vi "Save.vi"(8 "error in (no error)":errorcluster, 11 "Test Configs In":T1) -> (0 "error out":errorcluster, 3 "Test Configs Out":T1)   [LabVIEW 2015]
doc: "Save a test configuration XML file to the path chosen."
uses:
  Type Defs/Sequence Parameters Ref.ctl
  <vilib>/Utility/xml.llb/Write to XML File(string).vi
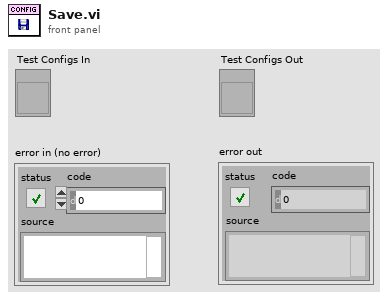
[diagram p1: front panel]
types:
  T1 = typedef "Sequence Parameters Ref.ctl" = refnum<vi>
  T2 = enum16{"open", "replace", "create", "open or create", "replace or create", "replace or create with confirmation"}
  T3 = typedef "Sequence Parameters.ctl" = cluster{"Test Name":string, "Target":T4, "Host IP Address":string, "Target IP Address":string, "Shared Variable Host":enum16{"Target", "Host"}, "Shared Variable Writer":enum16{"Target", "Host"}, "Variable Data Type":T5, "# of Variables per Library":u16, "Update Rate (Hz)":dbl, "Read Rate (Hz)":dbl, "Floor":u32, "Ceiling":u32, "Delta":u32}
  T4 = typedef "Target Type.ctl" = enum16{"cRIO-9012", "cRIO-9014", "cRIO-9022", "cRIO-9023", "cRIO-9024", "cRIO-9025", "cRIO-9068", "cRIO-9073", "cRIO-9074", "cRIO-9075", "cRIO-9076", "cRIO-9081", "cRIO-9082", "myRIO-1900", "myRIO-1950", "PXI-8101", "PXI-8115", "PXI-8119", "PXI-8820", "PXIe-8100", "PXIe-8101", "PXIe-8133", "PXIe-8135", "PXIe-8820", "sbRIO-9605", "sbRIO-9606", "sbRIO-9623", "sbRIO-9626", "sbRIO-9633", "sbRIO-9636", "Unlisted (Linux-RT)", "Unlisted (PharLap)", "Unlisted (VxWorks)", "Windows Target"}
  T5 = typedef "Variable Data Type.ctl" = enum16{"U8", "U16", "U32", "U64", "I8", "I16", "I32", "I64", "Single", "Double", "Boolean", "String"}
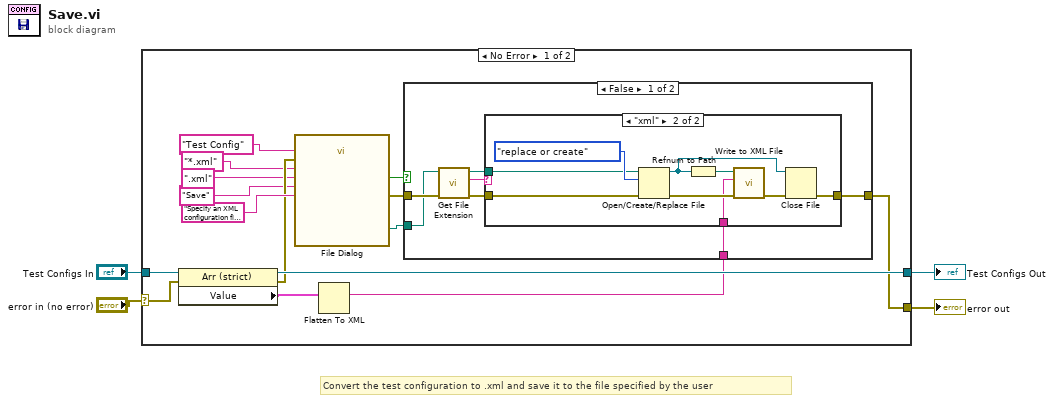
[diagram p0: block diagram]
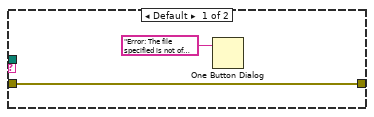
[diagram p2: hidden frame]
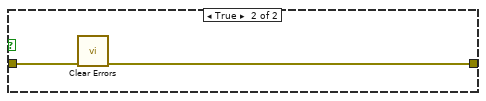
[diagram p3: hidden frame]
diagram:
  # "Convert the test configuration to .xml and save it to the file specified by the user"
  n1 = case shown="No Error" "error in (no error)" {
    selector: "error in (no error)" -> [w18 w40]
    tunnel: "Test Configs In" -> [w19 w41]
    tunnel: [w16 w41] -> w1
    tunnel: [w6 w40] -> w3
    frame No Error {
      n2 = property class="Arr (strict)"(reference=w19, error in=w18) -> (reference out=w16:T1, error out=w13:errorcluster, "Value"=w17:T3[])
      n3 = call "File Dialog"("prompt"="Specify an XML configuration file to create or replace", "button label"="Save", "default name"="Test Config", "error in"=w13, "pattern (all files)"="*.xml", "pattern label"=".xml" ("pattern (all files)")) -> ("selected path"=w10:path, "cancelled"=w12:bool, "error out"=w11:errorcluster)  [unwired: 6 in, 1 out]
      n4 = Flatten To XML(anything=w17) -> (xml string=w5:string)
      n5 = case shown="False" w12 {
        tunnel: w11 -> [w26 w39]
        tunnel: w10 -> [w25 _]
        tunnel: [w21 w38] -> w6
        tunnel: w5 -> [w20 _]
        frame False {
          n6 = call <vilib>:"Get File Extension.vi"("error in (no error)"=w26, "file"=w25) -> ("error out"=w23:errorcluster, "lowercase file extension"=w24:string, "dup file"=w22:path)  [unwired: 5 in, 2 out]
          n7 = case shown="\"xml\"" w24 {
            tunnel: w23 -> [w27 w33]
            tunnel: w22 -> [_ w32]
            tunnel: [w27 w30] -> w21
            tunnel: w20 -> [_ w29]
            frame Default {
              n8 = One Button Dialog(message="Error: The file specified is not of type (*.xml). Test configuration files must be saved using the XML schema.") -> ()  [unwired: 1 in, 1 out]
            }
            frame "xml" {
              n9 = Open/Create/Replace File(file path (use dialog)=w32, error in=w33, operation (0:open)=T2."replace or create") -> (refnum out=w31:refnum<file>, error out=w35:errorcluster)  [unwired: 3 in, 1 out]
              n10 = Refnum to Path(1:w31) -> (0:w36:path)
              n11 = call-poly <vilib>:"Write to XML File.vi"("error in (no error)"=w35, "XML Input"=w29, "XML File Path"=w36) -> ("error out"=w34:errorcluster)  [unwired: 6 in, 2 out]
              n12 = Close File(refnum=w31, error in=w34) -> (error out=w30:errorcluster)  [unwired: 1 out]
            }
          }
        }
        frame True {
          n13 = call <vilib>:"Clear Errors.vi"("error in (no error)"=w39) -> ("error out"=w38:errorcluster)  [unwired: 5 in, 1 out]
        }
      }
    }
    frame Error {
    }
  }
  "error out" <- w3
  "Test Configs Out" <- w1
